vi "Query Histogram.vi"(0 "VISA resource name":refnum<visa-resource-name>, 5 "Channel Name (1)":string="1", 9 "Bin Range (0: 8 A)":i32(ring) items=["8 A", "0.0039 A"], 11 "error in (no error)":errorcluster {"code" format="%.0x"}) -> (4 "VISA resource name out":refnum<visa-resource-name>, 6 "Current Bin Gain":dbl format="%^.3e", 8 "Current Bin Offset":dbl format="%^.3e", 10 "Current Bin Ranges":dbl format="%^.3e", 15 "error out":errorcluster {"code" format="%.0x"})   [LabVIEW 2016, in "Agilent N6700 Series.lvlib"]
doc: "Returns the current bin gain, bin offset, and bin range of the histogram.\n\n<b>Notes:</b>\n(1) This VI only applies to models N6781A and N6782A that have the Data Logger function installed.\n(2) This VI only applies to the N6705B and N6705C DC Power Analyzer."
uses:
  <instrlib>/Agilent N6700 Series/Agilent N6700 Series.lvlib
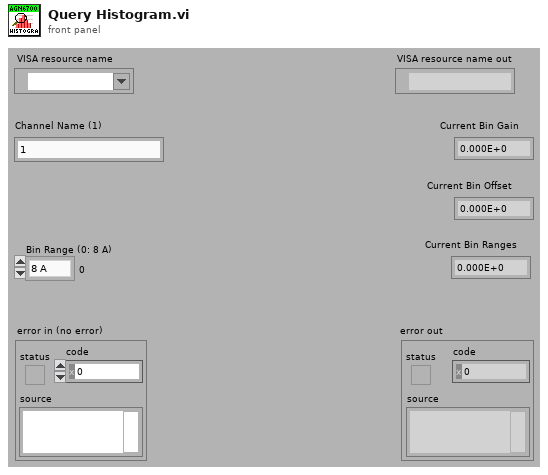
[diagram p1: front panel]
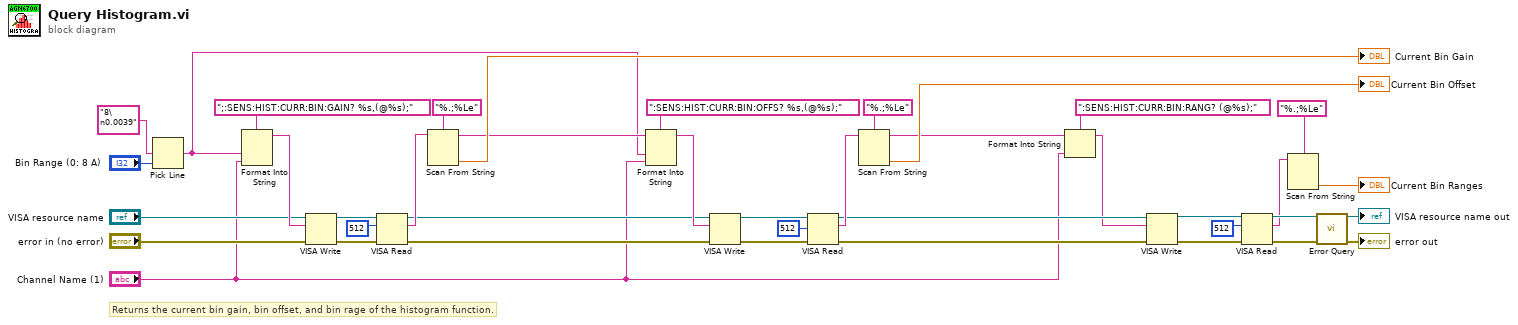
[diagram p0: block diagram]
diagram:
  # "Returns the current bin gain, bin offset, and bin rage of the histogram function."
  n1 = Pick Line(multi-line string="8\n0.0039", line index="Bin Range (0: 8 A)") -> (output string=w17:string)  [unwired: 1 in]
  n2 = Format Into String(format string=";:SENS:HIST:CURR:BIN:GAIN? %s,(@%s);", w17, "Channel Name (1)") -> (resulting string=w34:string)  [unwired: 2 in, 1 out]
  n3 = VISA Write(VISA resource name="VISA resource name", write buffer=w34, error in (no error)="error in (no error)") -> (VISA resource name out=w39:refnum<visa-resource-name>, error out=w38:errorcluster)  [unwired: 1 out]
  n4 = VISA Read(VISA resource name=w39, byte count=u32 512, error in (no error)=w38) -> (VISA resource name out=w11:refnum<visa-resource-name>, read buffer=w37:string, error out=w15:errorcluster)  [unwired: 1 out]
  n5 = Scan From String(format string="%.;%Le", input string=w37) -> (remaining string=w22:string, output 1=→"Current Bin Gain":dbl)  [unwired: 3 in, 2 out]
  n6 = Format Into String(format string=":SENS:HIST:CURR:BIN:OFFS? %s,(@%s);", initial string=w22, w17, "Channel Name (1)") -> (resulting string=w28:string)  [unwired: 1 in, 1 out]
  n7 = VISA Write(VISA resource name=w11, write buffer=w28, error in (no error)=w15) -> (VISA resource name out=w12:refnum<visa-resource-name>, error out=w16:errorcluster)  [unwired: 1 out]
  n8 = VISA Read(VISA resource name=w12, byte count=u32 512, error in (no error)=w16) -> (VISA resource name out=w10:refnum<visa-resource-name>, read buffer=w25:string, error out=w9:errorcluster)  [unwired: 1 out]
  n9 = Scan From String(format string="%.;%Le", input string=w25) -> (remaining string=w19:string, output 1=→"Current Bin Offset":dbl)  [unwired: 3 in, 2 out]
  n10 = Format Into String(format string=":SENS:HIST:CURR:BIN:RANG? (@%s);", initial string=w19, "Channel Name (1)") -> (resulting string=w6:string)  [unwired: 1 in, 1 out]
  n11 = VISA Write(VISA resource name=w10, write buffer=w6, error in (no error)=w9) -> (VISA resource name out=w2:refnum<visa-resource-name>, error out=w14:errorcluster)  [unwired: 1 out]
  n12 = VISA Read(VISA resource name=w2, byte count=u32 512, error in (no error)=w14) -> (VISA resource name out=w7:refnum<visa-resource-name>, read buffer=w5:string, error out=w8:errorcluster)  [unwired: 1 out]
  n13 = Scan From String(format string="%.;%Le", input string=w5) -> (output 1=→"Current Bin Ranges":dbl)  [unwired: 3 in, 3 out]
  n14 = call <instrlib>:"Error Query.vi"("VISA resource name"=w7, "error in (no error)"=w8) -> ("VISA resource name out"=→"VISA resource name out":refnum<visa-resource-name>, "error out"=→"error out":errorcluster)  [unwired: 10 in, 2 out]
